vi "Read System Setup Types .vi"(0 "ServerPath":path, 11 "Error In":errorcluster) -> (4 "Section Names":string[](array[string]), 15 "Error Out":errorcluster)   [LabVIEW 2013]
uses:
  <vilib>/Utility/config.llb/NI_LVConfig.lvlib
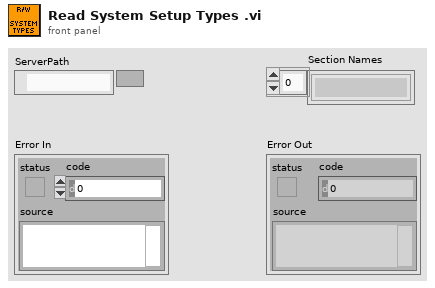
[diagram p1: front panel]
types:
  T1 = typedef "NI_LVConfig.lvlib/Config Data RefNum.ctl" = refnum<k1>
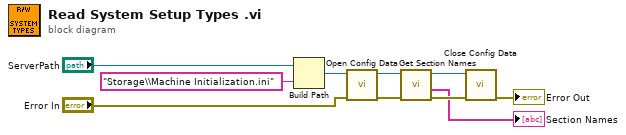
[diagram p0: block diagram]
diagram:
  n1 = Build Path(base path="ServerPath", name or relative path="Storage\\Machine Initialization.ini") -> (appended path=w9:path)
  n2 = call <vilib>:"Open Config Data.vi"("error in (no error)"="Error In", "configuration file path"=w9) -> ("error out"=w4:errorcluster, "refnum"=w5:T1)  [unwired: 7 in, 1 out]
  n3 = call <vilib>:"Get Section Names.vi"("error in (no error)"=w4, "refnum"=w5) -> ("error out"=w2:errorcluster, "section names"=→"Section Names":string[], "refnum out"=w3:T1)  [unwired: 7 in]
  n4 = call <vilib>:"Close Config Data.vi"("error in (no error)"=w2, "refnum"=w3) -> ("error out"=→"Error Out":errorcluster)  [unwired: 8 in, 1 out]
